vi "DraggingDresser.vi"() -> ()   [LabVIEW 2015]
panel:
  out "Force":dbl[](array[numeric])
  out "Angle for Minimum Force":i32 format="%.1f"
  in  "Coefficient of Kinetic Friction":dbl format="%.1f"
  out "Waveform Graph":dbl[](graph)
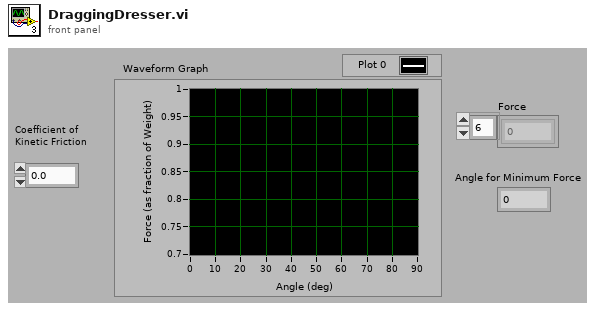
[diagram p1: front panel]
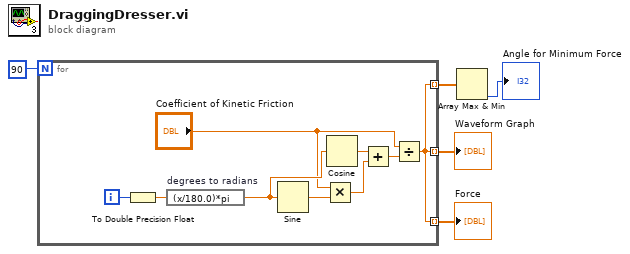
[diagram p0: block diagram]
diagram:
  n1 = for {
    N: 90 -> [_]
    tunnel: [w6] -> w4 mode=indexing
    tunnel: [w6] -> w2 mode=indexing
    tunnel: [w6] -> w1 mode=indexing
    i -> [w8]
    n2 = To Double Precision Float(number=w8) -> (double precision float=w7:dbl)
    n3 = expression code="(x/180.0)*pi" "degrees to radians"(w7) -> (w14:dbl)
    n4 = Sine(x=w14) -> (sin(x)=w12:dbl)
    n5 = Multiply(x="Coefficient of Kinetic Friction", y=w12) -> (x*y=w10:dbl)
    n6 = Cosine(x=w14) -> (cos(x)=w13:dbl)
    n7 = Add(x=w13, y=w10) -> (x+y=w9:dbl)
    n8 = Divide(x="Coefficient of Kinetic Friction", y=w9) -> (x/y=w6:dbl)
  }
  "Force" <- w4
  "Waveform Graph" <- w2
  n9 = Array Max & Min(array=w1) -> (min index (indices)=→"Angle for Minimum Force":i32)  [unwired: 3 out]
